vi "DriveAutoStraight.vi"(5 "D Gain":dbl=0.0004 format="%#_13g", 7 "P Gain":dbl=0.04 format="%#_13g", 8 "Initial Angle":dbl, 9 "Initial Time":timestamp, 10 "Target Distance (feet)":dbl, 11 "Directions":T1) -> (0 "Done?":bool, 2 "Right Motor Value":dbl, 3 "Left Motor Value":dbl)   [LabVIEW 2017]
uses:
  DriveAutoDirections.ctl
  SensorDataGlobal.vi
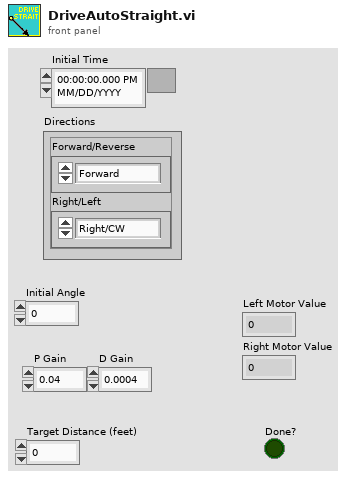
[diagram p1: front panel]
types:
  T1 = typedef "DriveAutoDirections.ctl" = cluster{"Forward/Reverse":enum16{"Forward", "Reverse"}, "Right/Left":enum16{"Right/CW", "Left/CCW"}}
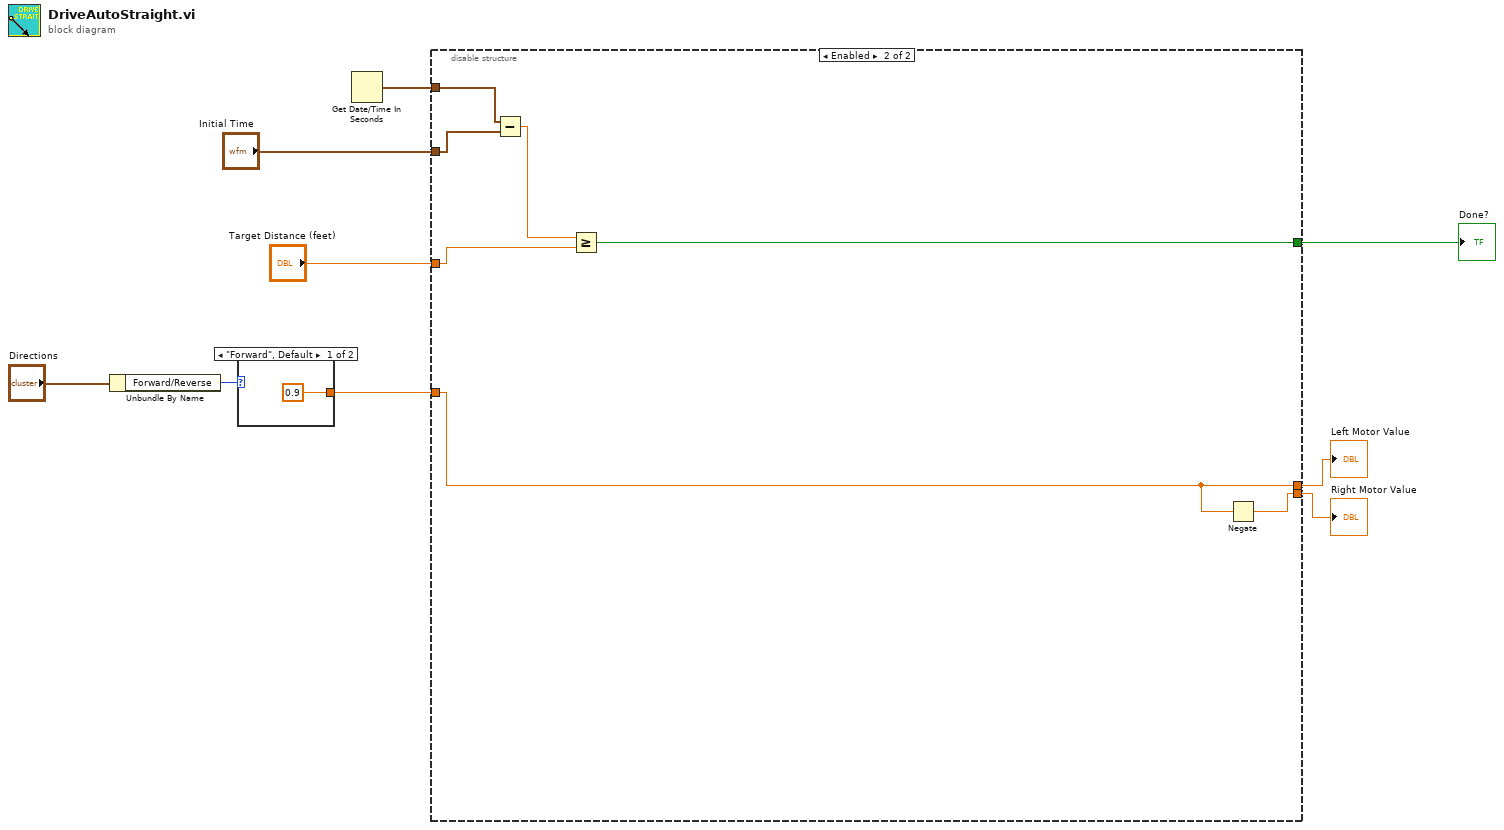
[diagram p0: block diagram]
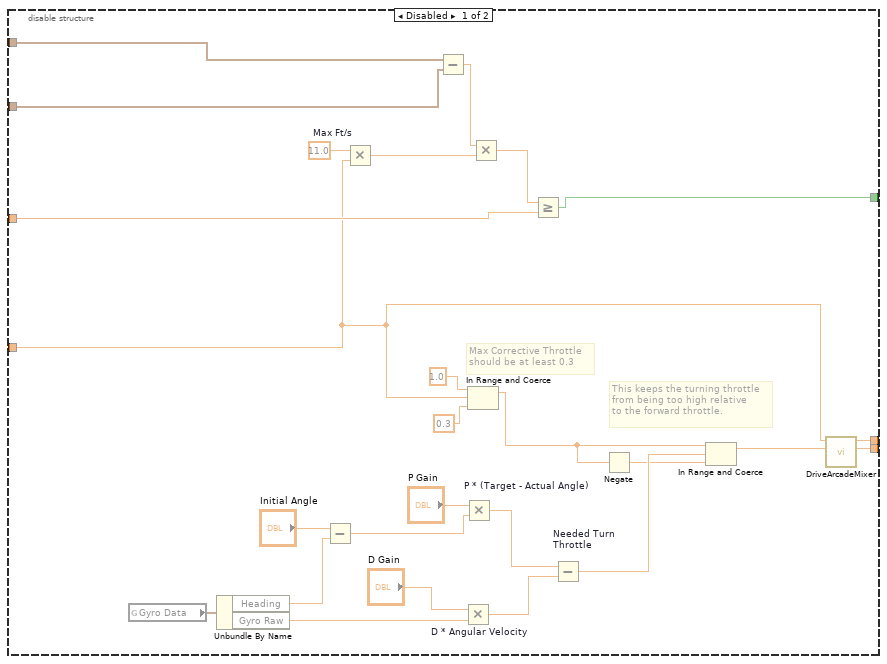
[diagram p2: hidden frame]
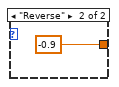
[diagram p3: hidden frame]
diagram:
  n1 = Unbundle By Name("Directions") -> ("Forward/Reverse"=w8:enum16{"Forward", "Reverse"})
  n2 = case shown="\"Forward\", Default" w8 {
    tunnel: [0.9 -0.9] -> w2
    frame "Forward", Default {
    }
    frame "Reverse" {
    }
  }
  n3 = Get Date/Time In Seconds() -> (seconds since 1Jan1904=w5:timestamp)
  n4 = disable-structure shown="Enabled" {
    disable-tunnel: [w22 w43] -> w7
    disable-tunnel: [w21 w44] -> w6
    disable-tunnel: w5 -> [w19 w42]
    disable-tunnel: "Initial Time" -> [w18 w41]
    disable-tunnel: "Target Distance (feet)" -> [w14 w39]
    disable-tunnel: w2 -> [w13 w43]
    disable-tunnel: [w12 w38] -> w1
    frame Disabled {
      w20 = 11.0  # Max Ft/s
      # "This keeps the turning throttle\nfrom being too high relative\nto the forward throttle."
      # "Max Corrective Throttle\nshould be at least 0.3"
      n5 = global read "SensorDataGlobal.vi" "Gyro Data"() -> (w29:cluster{"Heading":dbl, "Gyro Raw":dbl})
      n6 = Unbundle By Name(w29) -> ("Heading"=w26:dbl, "Gyro Raw"=w25:dbl)
      n7 = Subtract(x="Initial Angle", y=w26) -> (x-y=w37:dbl)
      n8 = Multiply(x=w20, y=w13) -> (x*y=w17:dbl)
      n9 = Subtract(x=w19, y=w18) -> (x-y=w16:dbl)
      n10 = Multiply "D * Angular Velocity"(x="D Gain", y=w25) -> (x*y=w35:dbl)
      n11 = Multiply "P * (Target - Actual Angle)"(x="P Gain", y=w37) -> (x*y=w36:dbl)
      n12 = In Range and Coerce(upper limit=1.0, x=w13, lower limit=0.3) -> (coerced(x)=w31:dbl)  [unwired: 1 out]
      n13 = Multiply(x=w16, y=w17) -> (x*y=w15:dbl)
      n14 = Greater Or Equal?(x=w15, y=w14) -> (x >= y?=w12:bool)
      n15 = Subtract "Needed Turn \nThrottle"(x=w36, y=w35) -> (x-y=w32:dbl)
      n16 = Negate(x=w31) -> (-x=w30:dbl)
      n17 = In Range and Coerce(upper limit=w31, x=w32, lower limit=w30) -> (coerced(x)=w23:dbl)  [unwired: 1 out]
      n18 = call "DriveArcadeMixer.vi"("X axis (turning) value"=w23, "Y axis (throttle) value"=w13) -> ("Right Motor Value"=w21:dbl, "Left Motor Value"=w22:dbl)  [unwired: 8 in]
    }
    frame Enabled {
      n19 = Subtract(x=w42, y=w41) -> (x-y=w40:dbl)
      n20 = Greater Or Equal?(x=w40, y=w39) -> (x >= y?=w38:bool)
      n21 = Negate(x=w43) -> (-x=w44:dbl)
    }
  }
  "Left Motor Value" <- w7
  "Right Motor Value" <- w6
  "Done?" <- w1
